vi "ExtractClass.vi"(7 "String":string, 11 "Array in":refnum<class "Class.lvclass">[](array[class])) -> (2 "ClassOut":refnum<class "Class.lvclass">, 3 "ArrayOut":refnum<class "Class.lvclass">[](array[class]))   [LabVIEW 2020, in "Mermaid.lvlib" / "Application.lvclass"]
uses:
  Application.lvclass
  _Class/Class.lvclass
  Application.lvclass/Application.ctl
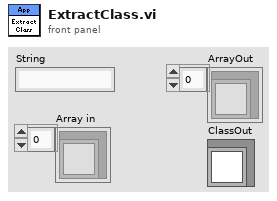
[diagram p1: front panel]
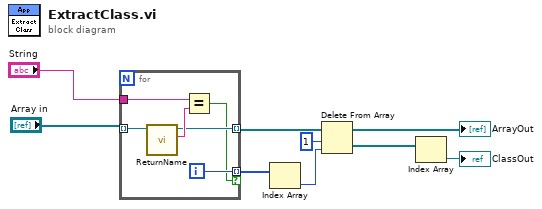
[diagram p0: block diagram]
diagram:
  n1 = for {
    tunnel: "Array in" -> [w15] mode=indexing
    tunnel: "String" -> [w13]
    tunnel: [w12] -> w3 mode=indexing
    tunnel: [w11] -> w8 mode=indexing if=w10
    i -> [w11]
    n2 = call-dynamic "ReturnName.vi"("Class in"=w15) -> ("Name"=w14:string, "Class out"=w12:refnum<class "Class.lvclass">)  [unwired: 8 in, 1 out]
    n3 = Equal?(x=w13, y=w14) -> (x = y?=w10:bool)
  }
  n4 = Index Array(array=w8) -> (element=w9:i32)  [unwired: 1 in]
  n5 = Delete From Array(array=w3, length=1, index=w9) -> (deleted portion=w2:refnum<class "Class.lvclass">[], array with subset deleted=→"ArrayOut":refnum<class "Class.lvclass">[])
  n6 = Index Array(array=w2) -> (element=→"ClassOut":refnum<class "Class.lvclass">)  [unwired: 1 in]
